vi "all_lines_in_frame.vi"(1 "focus mode?":bool, 2 "total number of lines per frame":u16, 3 "frame counter":u16) -> (0 "Numeric":u32)   [LabVIEW 2010]
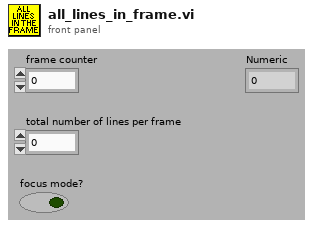
[diagram p1: front panel]
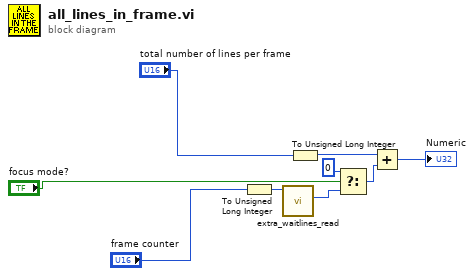
[diagram p0: block diagram]
diagram:
  n1 = To Unsigned Long Integer(number="frame counter") -> (unsigned 32bit integer=w1:u32)
  n2 = call "extra_waitlines_read.vi"("address extra waitlines IN"=w1) -> ("extra waitline data"=w2:u32)  [unwired: 9 in, 1 out]
  n3 = To Unsigned Long Integer(number="total number of lines per frame") -> (unsigned 32bit integer=w6:u32)
  n4 = Select(t=u32 0, s="focus mode?", f=w2) -> (s? t:f=w3:u32)
  n5 = Add(x=w6, y=w3) -> (x+y=→"Numeric":u32)
